vi "Main.vi"() -> ()   [LabVIEW 2018]
doc: "The myRIO Project template acquires acceleration data from the onboard accelerometer and displays the changes of acceleration values in a waveform chart."
uses:
  <vilib>/myRIO/Instrument Drivers/Onboard IO/AI/typedefs/AI Reference.ctl
  <vilib>/myRIO/Common/Instrument Driver Framework/Utilities/typedefs/myRIO Generic Hardware Reference.ctl
  <vilib>/myRIO/Common/Instrument Driver Framework/Utilities/typedefs/Hardware Version Enum.ctl
  <vilib>/myRIO/Common/Instrument Driver Framework/Utilities/typedefs/myRIO v1.0 Reference.ctl
  <vilib>/myRIO/Common/Instrument Driver Framework/Utilities/typedefs/Generic FPGA Reference.ctl
  <vilib>/myRIO/Common/Instrument Driver Framework/myRIO v1.0/AI/typedefs/AI Channels List.ctl
  <vilib>/myRIO/Common/Instrument Driver Framework/myRIO v1.0/AI/typedefs/AI Channels Enum.ctl
  <vilib>/myRIO/Common/Instrument Driver Framework/Utilities/typedefs/Analog Scaling Constants List.ctl
  <vilib>/myRIO/Common/Instrument Driver Framework/Utilities/typedefs/Analog Scaling Constants.ctl
  <vilib>/userdefined/High Color/nirio_resource_hc.ctl
  <vilib>/myRIO/Instrument Drivers/Onboard IO/PWM/typedefs/PWM Reference.ctl
  <vilib>/myRIO/Common/Instrument Driver Framework/myRIO v1.0/PWM/typedefs/PWM Channels Enum.ctl
  <vilib>/myRIO/Instrument Drivers/Onboard IO/PWM/typedefs/PWM Configuration.ctl
  <vilib>/myRIO/Common/Instrument Driver Framework/myRIO v1.0/AI/vis/myRIO v1.1 Open AI.vi
  <vilib>/myRIO/Common/Instrument Driver Framework/myRIO v1.0/PWM/vis/myRIO v1.1 Open PWM.vi
  <vilib>/myRIO/Common/Instrument Driver Framework/Utilities/vis/Validate Channels.vi
  <vilib>/myRIO/Common/Instrument Driver Framework/myRIO v1.0/AI/vis/myRIO v1.0 Reserve AI.vi
  <vilib>/myRIO/Common/Instrument Driver Framework/myRIO v1.0/PWM/vis/myRIO v1.0 Reserve PWM.vi
  <vilib>/myRIO/Common/Instrument Driver Framework/myRIO v1.0/PWM/vis/myRIO v1.0 Close PWM.vi
  <vilib>/myRIO/Common/Instrument Driver Framework/myRIO v1.0/AI/vis/myRIO v1.0 Close AI.vi
  <vilib>/myRIO/Common/Instrument Driver Framework/myRIO v1.0/UART/vis/myRIO v1.0 Close UART.vi
  <vilib>/myRIO/Common/Instrument Driver Framework/myRIO v1.0/AI/vis/myRIO v1.0 Build MUX Configuration AI.vi
  <vilib>/myRIO/Common/Instrument Driver Framework/myRIO v1.0/Resource Manager/vis/myRIO v1.0 Reserve Channel List.vi
  <vilib>/myRIO/Common/Instrument Driver Framework/myRIO v1.0/PWM/vis/myRIO v1.0 Build MUX Configuration PWM.vi
  <vilib>/myRIO/Common/Instrument Driver Framework/myRIO v1.0/PWM/vis/myRIO v1.0 Unreserve PWM.vi
  <vilib>/myRIO/Common/Instrument Driver Framework/myRIO v1.0/AI/vis/myRIO v1.0 Unreserve AI.vi
  <vilib>/myRIO/Common/Instrument Driver Framework/myRIO v1.0/Resource Manager/vis/myRIO v1.0 Reserve Channel.vi
  <vilib>/myRIO/Common/Instrument Driver Framework/myRIO v1.0/Resource Manager/vis/myRIO v1.0 Unreserve Channel.vi
  <vilib>/myRIO/Common/Instrument Driver Framework/myRIO v1.0/Resource Manager/vis/myRIO v1.0 Create Configuration List.vi
  <vilib>/myRIO/Common/Instrument Driver Framework/myRIO v1.0/Resource Manager/vis/myRIO v1.0 Unreserve Channel List.vi
  <vilib>/myRIO/Common/Instrument Driver Framework/myRIO v1.0/Resource Manager/vis/myRIO v1.0 Build Mutex Name.vi
  <vilib>/Utility/VariantDataType/GetNumericInfo.vi
  <vilib>/Utility/error.llb/Error Cluster From Error Code.vi
  <vilib>/myRIO/Common/Instrument Driver Framework/myRIO v1.0/myRIO v1.1 Open.vi
  <vilib>/myRIO/Common/Instrument Driver Framework/myRIO v1.0/AI/vis/myRIO v1.0 Get Scaling Constants AI.vi
  <vilib>/myRIO/Common/Instrument Driver Framework/Utilities/vis/IO Manager.vi
  <vilib>/myRIO/Common/Instrument Driver Framework/Utilities/vis/Configuration Manager.vi
  <vilib>/myRIO/Common/Instrument Driver Framework/myRIO v1.0/myRIO v1.0 Close.vi
  <vilib>/myRIO/Common/Instrument Driver Framework/myRIO v1.0/Resource Manager/vis/myRIO v1.0 Configure IO.vi
  <vilib>/myRIO/Common/Instrument Driver Framework/myRIO v1.0/PWM/vis/myRIO v1.0 Write PWM.vi
  <vilib>/myRIO/Common/Instrument Driver Framework/myRIO v1.0/AI/vis/myRIO v1.0 Read AI.vi
  <vilib>/myRIO/Common/Instrument Driver Framework/myRIO v1.0/PWM/vis/myRIO v1.0 Shutdown PWM.vi
  <vilib>/myRIO/Common/Instrument Driver Framework/Utilities/vis/FPGA Ref Manager.vi
  <vilib>/myRIO/Common/Instrument Driver Framework/myRIO v1.0/myRIO v1.0 Reset FPGA.vi
  <vilib>/myRIO/Common/Instrument Driver Framework/myRIO v1.0/IRQ/vis/myRIO v1.0 IRQ Info FGV.vi
  <vilib>/myRIO/Common/Instrument Driver Framework/myRIO v1.0/IRQ/vis/myRIO v1.0 Timer IRQ Info FGV.vi
  <vilib>/myRIO/Common/Instrument Driver Framework/myRIO v1.0/IRQ/vis/myRIO v1.0 ISR Agent.vi
  <vilib>/myRIO/Instrument Drivers/Onboard IO/AI/vis/myRIO AI Open.xnode
  <vilib>/myRIO/Instrument Drivers/Onboard IO/PWM/vis/myRIO PWM Open.xnode
  <vilib>/myRIO/Instrument Drivers/Utilities/Utilities.lvlib
  <vilib>/myRIO/Instrument Drivers/Onboard IO/PWM/PWM.lvlib
  <vilib>/myRIO/Instrument Drivers/Onboard IO/AI/AI.lvlib
panel:
  out "Batteri tilbage (%)":dbl
  out "Mean 50":dbl format="%0.2f"
  out "Mean 100":dbl format="%0.2f"
  in  "Threshold forskel":dbl=0.02 format="%#_13g"
  in  "Stop Button 2":bool
  in  "Hz 2":dbl
  in  "DC 2":dbl format="%#_13g"
  out "Duty Cycle":dbl
  in  "Boost":bool
  out "Waveform Chart":dbl(graph)
  out "Målt ampere":dbl
  in  "Frequency [Hz]":dbl=200.0
  in  "Duty Cycle":dbl=100.0
  out "error out":errorcluster
  in  "Stop":bool
  # "WIRING:\nBrun = GND\nOrange = PWM (A/DIO8)"
  # "100 = max\n50 = 0\n0 = -max"
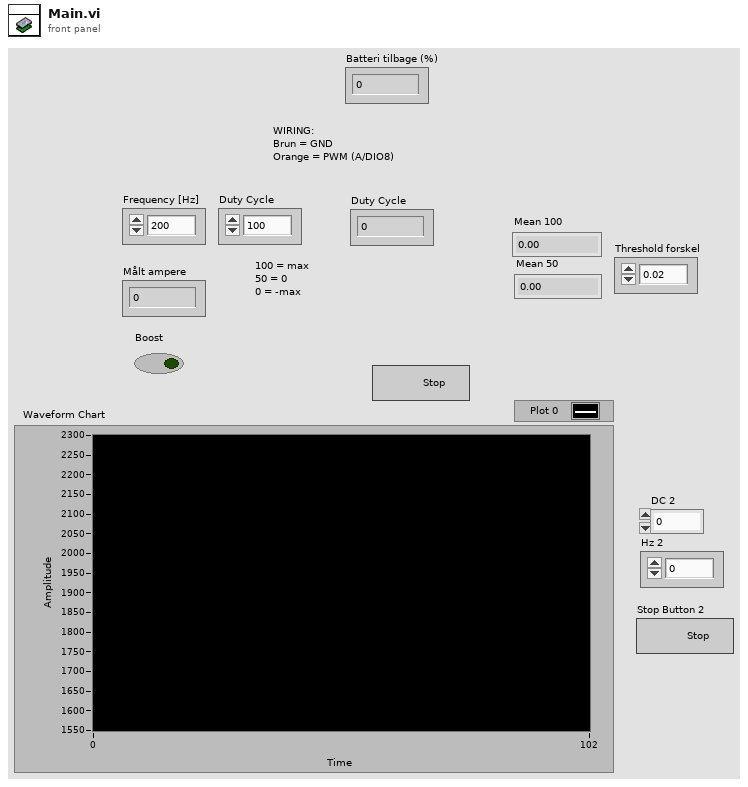
[diagram p1: front panel]
types:
  T1 = typedef "nirio_resource_hc.ctl" = tag
  T2 = typedef "Hardware Version Enum.ctl" = enum16{"Unknown", "myRIO-1900", "myRIO-1950", "roboRIO", "NI ELVIS RIO CM", "ELVIS III"}
  T3 = typedef "AI.lvlib/AI Reference.ctl" = cluster{"myRIO Reference":T4, "AI Channels List":T7, "AI Scaling Constants List":T9}
  T4 = typedef "myRIO Generic Hardware Reference.ctl" = cluster{"myRIO Model":T2, "myRIO Hardware Reference":T5}
  T5 = typedef "myRIO v1.0 Reference.ctl" = cluster{"Generic FPGA Reference":T6, "Allow multiple opens":bool}
  T6 = typedef "Generic FPGA Reference.ctl" = refnum<k20>
  T7 = typedef "AI Channels List.ctl" = T8[]
  T8 = typedef "AI Channels Enum.ctl" = enum16{"Not Connected", "AudioIn/Left", "AudioIn/Right", "C/AI0", "C/AI1", "A/AI0", "A/AI1", "A/AI2", "A/AI3", "A/AI4", "A/AI5", "A/AI6", "A/AI7", "B/AI0", "B/AI1", "B/AI2", "B/AI3", "B/AI4", "B/AI5", "B/AI6", "B/AI7", "AI/AI0", "AI/AI1", "AI/AI2", "AI/AI3", "A/AI0 (DIFF)", "A/AI1 (DIFF)", "A/AI2 (DIFF)", "A/AI3 (DIFF)", "B/AI0 (DIFF)", "B/AI1 (DIFF)", "B/AI2 (DIFF)", "B/AI3 (DIFF)"}
  T9 = typedef "Analog Scaling Constants List.ctl" = T10[]
  T10 = typedef "Analog Scaling Constants.ctl" = cluster{"LSB Weight (Volts)":dbl, "Offset (Volts)":dbl, "Signed?":bool}
  T11 = typedef "PWM.lvlib/PWM Reference.ctl" = cluster{"myRIO Reference":T4, "PWM Channels Enum":T12, "PWM Configuration":T13}
  T12 = typedef "PWM Channels Enum.ctl" = enum16{"Not Connected", "C/PWM0", "C/PWM1", "A/PWM0", "A/PWM1", "A/PWM2", "A/PWM3", "A/PWM4", "A/PWM5", "A/PWM6", "A/PWM7", "A/PWM8", "A/PWM9", "A/PWM10", "A/PWM11", "A/PWM12", "A/PWM13", "A/PWM14", "A/PWM15", "A/PWM16", "A/PWM17", "A/PWM18", "A/PWM19", "B/PWM0", "B/PWM1", "B/PWM2", "B/PWM3", "B/PWM4", "B/PWM5", "B/PWM6", "B/PWM7", "B/PWM8", "B/PWM9", "B/PWM10", "B/PWM11", "B/PWM12", "B/PWM13", "B/PWM14", "B/PWM15", "B/PWM16", "B/PWM17", "B/PWM18", "B/PWM19", "PWM/PWM0", "PWM/PWM1", "PWM/PWM2", "PWM/PWM3", "PWM/PWM4", "PWM/PWM5", "PWM/PWM6", "PWM/PWM7", "PWM/PWM8", "PWM/PWM9"}
  T13 = typedef "PWM.lvlib/PWM Configuration.ctl" = cluster{"Frequency":dbl, "Duty Cycle":dbl}
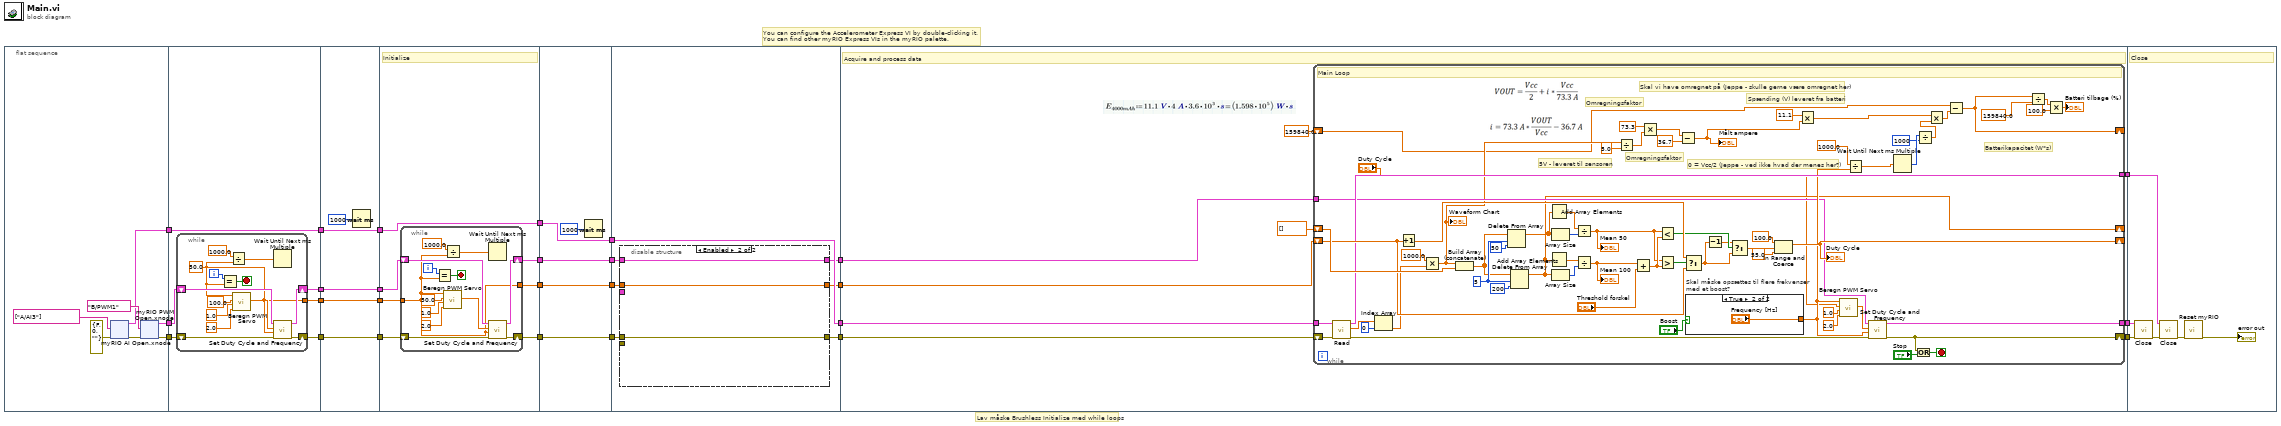
[diagram p0: block diagram]
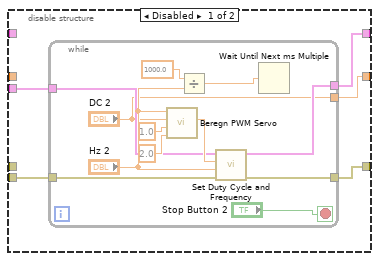
[diagram p2: hidden frame]
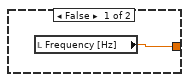
[diagram p3: hidden frame]
diagram:
  # "Lav måske Brushless Initialize med while loops"
  # "You can configure the Accelerometer Express VI by double-clicking it.\nYou can find other myRIO Express VIs in the myRIO palette."
  n1 = flat-sequence {
    tunnel: [w31] -> w25
    tunnel: [w30] -> w22
    tunnel: [w27] -> w14
    tunnel: w25 -> [w73]
    tunnel: [w73] -> w24
    tunnel: w22 -> [w72]
    tunnel: [w71] -> w21
    tunnel: [w70] -> w15
    tunnel: w14 -> [w69]
    tunnel: [w68] -> w12
    tunnel: w24 -> [w90]
    tunnel: [w90] -> w23
    tunnel: w21 -> [w89]
    tunnel: [w89] -> w20
    tunnel: [w88] -> w16
    tunnel: w15 -> [w88]
    tunnel: [w87] -> w13
    tunnel: w12 -> [w87]
    tunnel: w23 -> [w98]
    tunnel: [w98] -> w17
    tunnel: w20 -> [w95]
    tunnel: w16 -> [w97]
    tunnel: w13 -> [w96]
    tunnel: [w92] -> w11
    tunnel: [w94] -> w6
    tunnel: [w93] -> w5
    tunnel: w17 -> [w116]
    tunnel: [w116] -> w4
    tunnel: w11 -> [w113]
    tunnel: w6 -> [w112]
    tunnel: w5 -> [w114]
    tunnel: [w114] -> w3
    tunnel: [w113] -> w2
    tunnel: [w112] -> w1
    tunnel: [w121] -> w10
    tunnel: w4 -> [w123]
    tunnel: [w123] -> w9
    tunnel: [w122] -> w8
    tunnel: [w120] -> w7
    tunnel: w3 -> [w119]
    tunnel: w2 -> [w118]
    tunnel: w1 -> [w117]
    tunnel: w10 -> [w152]
    tunnel: [w151] -> w26
    tunnel: w9 -> [w150]
    tunnel: w8 -> [w149]
    tunnel: [w148] -> w19
    tunnel: [w147] -> w18
    tunnel: w7 -> [w146]
    tunnel: w26 -> [w224]
    tunnel: w19 -> [w221]
    tunnel: w18 -> [w220]
    frame #0 {
      n2 = xnode "myRIO AI Open.xnode"("error in (no error)"=errorcluster {"status"=FALSE, "code"=0, "source"=""}, "Channel Names"=tag[] ["A/AI3"]) -> ("error out"=w28:errorcluster, "AI Ref Out"=w31:T3)  [unwired: 1 in]
      n3 = xnode "myRIO PWM Open.xnode"("error in (no error)"=w28, "Channel Name"=tag "B/PWM1") -> ("error out"=w27:errorcluster, "PWM Ref Out"=w30:T11)  [unwired: 1 in]
    }
    frame #1 {
      n4 = while {
        tunnel: [w76] -> w70
        shift-right: [w81] -> w71
        shift-left: w72 -> [w83]
        shift-right: [w79] -> w68
        shift-left: w69 -> [w80]
        i -> [w78]
        stop <- w74 stop-if-true
        w76 = 50.0 ("Frequency [Hz]")
        n5 = Equal?(x=w78, y=w76) -> (x = y?=w74:bool)
        n6 = Divide(x=1000.0, y=w76) -> (x/y=w77:dbl)
        n7 = call "Beregn PWM Servo.vi"("Max (ms puls bredde)"=2.0, "Min (ms puls bredde)"=1.0, "Duty Cycle"=100.0, "Frekvens"=w76) -> ("Output Dutycycle til PWM Servo"=w82:dbl)  [unwired: 7 in]
        n8 = Wait Until Next ms Multiple(millisecond multiple=w77) -> ()  [unwired: 1 out]
        n9 = call <vilib>:"Set Duty Cycle and Frequency.vi"("error in (no error)"=w80, "Frequency [Hz]"=w76, "Duty Cycle"=w82, "PWM Ref In"=w83) -> ("error out"=w79:errorcluster, "PWM Ref Out"=w81:T11)  [unwired: 5 in]
      }
    }
    frame #2 {
      n10 = Wait (ms)(milliseconds to wait=u32 1000) -> ()  [unwired: 1 out]
    }
    frame #3 {
      # "Initialize"
      n11 = while {
        tunnel: [w99] -> w93
        shift-right: [w106] -> w94
        shift-left: w95 -> [w108]
        shift-right: [w104] -> w92
        shift-left: w96 -> [w105]
        tunnel: w97 -> [w99]
        i -> [w103]
        stop <- w100 stop-if-true
        n12 = Equal?(x=w103, y=w99) -> (x = y?=w100:bool)
        n13 = call "Beregn PWM Servo.vi"("Max (ms puls bredde)"=2.0, "Min (ms puls bredde)"=1.0, "Duty Cycle"=50.0, "Frekvens"=w99) -> ("Output Dutycycle til PWM Servo"=w107:dbl)  [unwired: 7 in]
        n14 = Divide(x=1000.0, y=w99) -> (x/y=w102:dbl)
        n15 = Wait Until Next ms Multiple(millisecond multiple=w102) -> ()  [unwired: 1 out]
        n16 = call <vilib>:"Set Duty Cycle and Frequency.vi"("error in (no error)"=w105, "Frequency [Hz]"=w99, "Duty Cycle"=w107, "PWM Ref In"=w108) -> ("error out"=w104:errorcluster, "PWM Ref Out"=w106:T11)  [unwired: 5 in]
      }
    }
    frame #4 {
      n17 = Wait (ms)(milliseconds to wait=u32 1000) -> ()  [unwired: 1 out]
    }
    frame #5 {
      n18 = disable-structure shown="Enabled" {
        disable-tunnel: _ -> [w128 _]
        disable-tunnel: [w127 w141] -> w122
        disable-tunnel: _ -> [w126 _]
        disable-tunnel: [w125 w142] -> w121
        disable-tunnel: [w124 w143] -> w120
        disable-tunnel: w119 -> [_ w143]
        disable-tunnel: w118 -> [_ w142]
        disable-tunnel: w117 -> [_ w141]
        frame Disabled {
          n19 = while {
            tunnel: w128 -> [w133]
            tunnel: [w132] -> w127
            tunnel: [w134] -> w125
            tunnel: w126 -> [w130]
            tunnel: ["DC 2"] -> w124
            stop <- "Stop Button 2" stop-if-true
            n20 = call "Beregn PWM Servo.vi"("Max (ms puls bredde)"=2.0, "Min (ms puls bredde)"=1.0, "Duty Cycle"="DC 2", "Frekvens"="Hz 2") -> ("Output Dutycycle til PWM Servo"=w135:dbl)  [unwired: 7 in]
            n21 = Divide(x=1000.0, y="Hz 2") -> (x/y=w138:dbl)
            n22 = call <vilib>:"Set Duty Cycle and Frequency.vi"("error in (no error)"=w130, "Frequency [Hz]"="Hz 2", "Duty Cycle"=w135, "PWM Ref In"=w133) -> ("error out"=w134:errorcluster, "PWM Ref Out"=w132:T11)  [unwired: 5 in]
            n23 = Wait Until Next ms Multiple(millisecond multiple=w138) -> ()  [unwired: 1 out]
          }
        }
        frame Enabled {
        }
      }
    }
    frame #6 {
      # "Acquire and process data"
      n24 = while {
        shift-right: [w195] -> w151
        shift-left: w152 -> [w200]
        shift-right: [w180] -> _
        shift-left: dbl[] [] -> [w213]
        shift-right: [w201] -> _
        shift-left: w146 -> [w208]
        tunnel: w150 -> [w199]
        tunnel: w149 -> [w188]
        tunnel: [w194] -> w148
        tunnel: [w193] -> w147
        shift-right: [w158] -> _
        shift-left: 159840.0 -> [w159]
        stop <- w216 stop-if-true
        w187 = 5 ("length")
        # "Batterikapacitet (W*s)"
        # "Spænding (V) leveret fra batteri"
        # "Omregningsfaktor"
        # "Omregningsfaktor"
        # "5V - leveret til sensoren"
        # "Skal vi have omregnet på (Jeppe - skulle gerne være omregnet her)"
        # "0 = Vcc/2 (Jeppe - ved ikke hvad der menes her?)"
        # "Main Loop"
        n25 = call <vilib>:"Read.vi"("error in (no error)"=w200, "AI Ref In"=w199) -> ("error out"=w196:errorcluster, "Values"=w198:dbl[], "AI Ref Out"=w193:T3)  [unwired: 7 in]
        n26 = Index Array(array=w198, index=0) -> (element=w174:dbl)
        n27 = Increment(x=w208) -> (x+1=w210:dbl)
        n28 = Multiply(x=1000.0, y=w174) -> (x*y=w172:dbl)
        "Waveform Chart" <- w172
        n29 = Build Array (concatenate)(w172, w213) -> (w185:dbl[])
        n30 = Delete From Array(array=w185, length=w187, index=50) -> (array with subset deleted=w176:dbl[])  [unwired: 1 out]
        n31 = Delete From Array(array=w185, length=w187, index=200) -> (array with subset deleted=w180:dbl[])  [unwired: 1 out]
        n32 = Add Array Elements(numeric array=w176) -> (sum=w177:dbl)
        n33 = Add Array Elements(numeric array=w180) -> (sum=w182:dbl)
        n34 = Array Size(array=w176) -> (size(s)=w178:i32)
        n35 = Array Size(array=w180) -> (size(s)=w181:i32)
        n36 = Divide(x=w177, y=w178) -> (x/y=w175:dbl)
        "Mean 50" <- w175
        n37 = Divide(x=w182, y=w181) -> (x/y=w179:dbl)
        "Mean 100" <- w179
        n38 = Divide(x=w172, y=5.0) -> (x/y=w170:dbl)
        n39 = Add(x=w179, y="Threshold forskel") -> (x+y=w184:dbl)
        n40 = Multiply(x=73.3, y=w170) -> (x*y=w168:dbl)
        n41 = Less?(x=w175, y=w184) -> (x < y?=w207:bool)
        n42 = Greater?(x=w175, y=w184) -> (0:w209:bool)
        n43 = Subtract(x=w168, y=36.7) -> (x-y=w165:dbl)
        "Målt ampere" <- w165
        n44 = Select(t=w210, s=w209, f=w208) -> (s? t:f=w206:dbl)
        n45 = case "Skal måske opsættes til flere frekvenser\nmed et boost?" shown="True" "Boost" {
          tunnel: [w218 "Frequency [Hz]"] -> w190
          frame False {
            n46 = local read "Frequency [Hz]"() -> (w218:dbl)
          }
          frame True {
          }
        }
        n47 = Decrement(x=w206) -> (x-1=w205:dbl)
        n48 = Select(t=w205, s=w207, f=w206) -> (s? t:f=w204:dbl)
        n49 = In Range and Coerce(upper limit=100.0, x=w204, lower limit=55.0) -> (coerced(x)=w201:dbl)  [unwired: 1 out]
        "Duty Cycle" <- w201
        n50 = Multiply(x=11.1, y=w165) -> (x*y=w164:dbl)
        n51 = call "Beregn PWM Servo.vi"("Max (ms puls bredde)"=2.0, "Min (ms puls bredde)"=1.0, "Duty Cycle"="Duty Cycle", "Frekvens"=w190) -> ("Output Dutycycle til PWM Servo"=w197:dbl)  [unwired: 7 in]
        n52 = Divide(x=1000.0, y=w190) -> (x/y=w191:dbl)
        n53 = call <vilib>:"Set Duty Cycle and Frequency.vi"("error in (no error)"=w196, "Frequency [Hz]"=w190, "Duty Cycle"=w197, "PWM Ref In"=w188) -> ("error out"=w195:errorcluster, "PWM Ref Out"=w194:T11)  [unwired: 5 in]
        n54 = Wait Until Next ms Multiple(millisecond multiple=w191) -> (millisecond timer value=w163:u32)
        n55 = Or(x=w195, y="Stop") -> (x .or. y?=w216:bool)
        n56 = Divide(x=w163, y=u32 1000) -> (x/y=w161:dbl)
        n57 = Multiply(x=w164, y=w161) -> (x*y=w160:dbl)
        n58 = Subtract(x=w159, y=w160) -> (x-y=w158:dbl)
        n59 = Divide(x=w158, y=159840.0) -> (x/y=w156:dbl)
        n60 = Multiply(x=w156, y=100.0) -> (x*y=→"Batteri tilbage (%)":dbl)
      }
    }
    frame #7 {
      # "Close"
      n61 = call <vilib>:"Close.vi"("error in (no error)"=w224, "PWM Ref In"=w221) -> ("error out"=w223:errorcluster)  [unwired: 9 in]
      n62 = call <vilib>:"Close.vi"("error in (no error)"=w223, "AI Ref In"=w220) -> ("error out"=w222:errorcluster)  [unwired: 9 in]
      n63 = call <vilib>:"Reset myRIO.vi"("error in (no error)"=w222) -> ("error out"=→"error out":errorcluster)  [unwired: 10 in]
    }
  }
